vi "Actuonix LAX breaker actuator TEST.vi"(3 "error in (no error)":errorcluster) -> (5 "Breaker State":bool, 7 "position":dbl, 10 "error out":errorcluster)   [LabVIEW 2019]
panel:
  in  "buttonRESET":bool
  in  "buttonOFF":bool
  in  "buttonON":bool
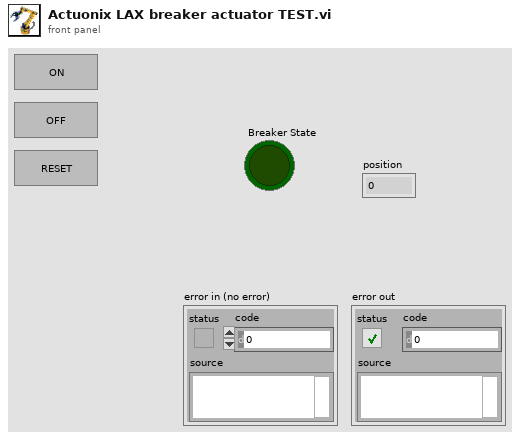
[diagram p1: front panel]
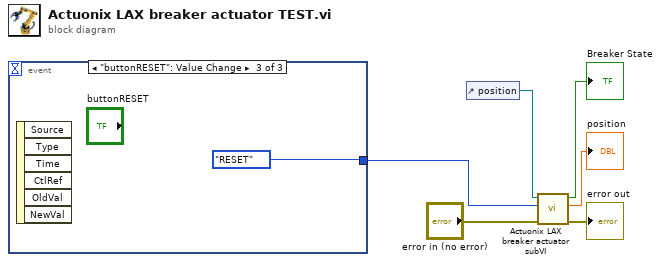
[diagram p0: block diagram]
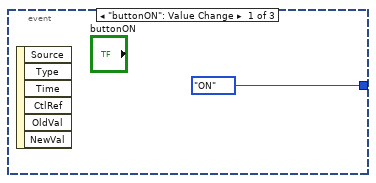
[diagram p2: hidden frame]
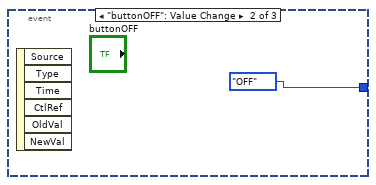
[diagram p3: hidden frame]
diagram:
  n1 = event shown="[2] \"buttonRESET\": Value Change" {
    selector: _ -> [_ _ _]
    dyn-events: _ -> [_ _ _]
    timeout: _ -> [_ _ _]
    tunnel: [enum16{"OFF", "ON", "RESET"}."ON" ("actionEnum") enum16{"OFF", "ON", "RESET"}."OFF" ("actionEnum") enum16{"OFF", "ON", "RESET"}."RESET" ("actionEnum")] -> w1
    event "buttonON": Value Change {
      n2 = event-data() -> ()  [unwired: 1 in, 6 out]
    }
    event "buttonOFF": Value Change {
      n3 = event-data() -> ()  [unwired: 1 in, 6 out]
    }
    event "buttonRESET": Value Change {
      n4 = event-data() -> ()  [unwired: 1 in, 6 out]
    }
  }
  n5 = control-ref of="position"() -> (w5:refnum<vi>)
  n6 = call "Actuonix LAX breaker actuator subVI.vi"("error in (no error)"="error in (no error)", "actionEnum"=w1, "Digital in"=w5) -> ("error out"=→"error out":errorcluster, "position"=→"position":dbl, "Breaker State"=→"Breaker State":bool)  [unwired: 6 in]
